vi "Get_File_Name.vi"() -> (0 "File Name":path)   [LabVIEW 2018]
uses:
  <vilib>/Rock Robotics/Network Tables/NT Read String.vi
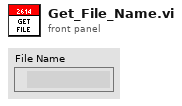
[diagram p1: front panel]
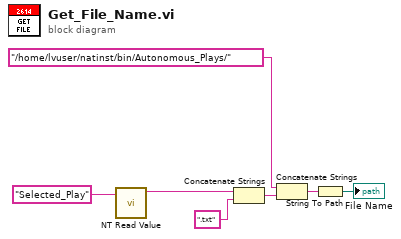
[diagram p0: block diagram]
diagram:
  n1 = call-poly <vilib>:"NT Read Value.vi"("Name"="Selected_Play") -> ("String"=w2:string)  [unwired: 9 in, 1 out]
  n2 = Concatenate Strings(w2, ".txt" ("string")) -> (w4:string)
  n3 = Concatenate Strings("/home/lvuser/natinst/bin/Autonomous_Plays/" ("string"), w4) -> (w7:string)
  n4 = String To Path(string=w7) -> (path=→"File Name":path)
